vi "neo_sebesseg.vi"(7 "Jobb":dbl(slide) scale=-5.0..5.0, 8 "error in (no error)":errorcluster, 9 "Bal":dbl(slide) scale=-5.0..5.0, 10 "new reference in":refnum<k24>) -> (0 "error out":errorcluster, 2 "vissza":bool, 3 ".NET Refnum out":refnum<k24>)   [LabVIEW 2012]
uses:
  RosBridgeDotNet.dll
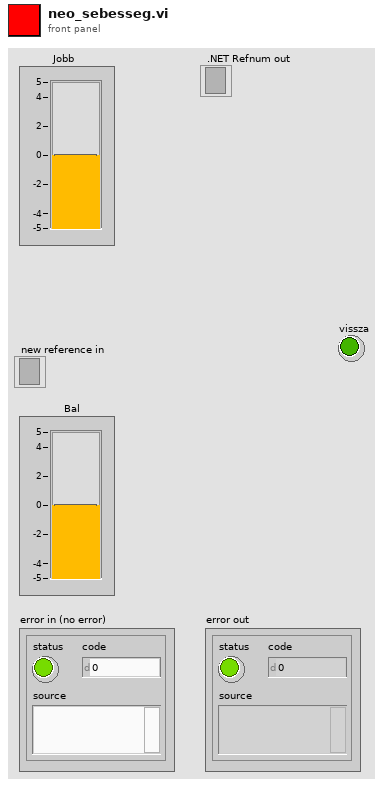
[diagram p1: front panel]
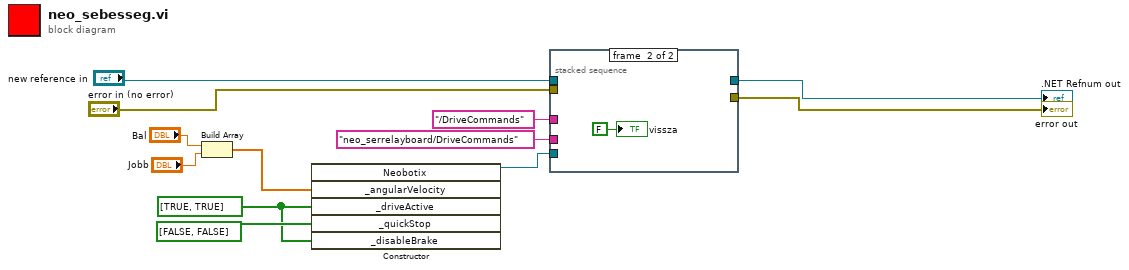
[diagram p0: block diagram]
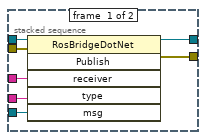
[diagram p2: hidden frame]
diagram:
  w8 = bool[] [TRUE, TRUE] ("_driveActive")
  n1 = Build Array("Bal", "Jobb") -> (w10:dbl[])
  n2 = constructor class="RosBridgeDotNet+Neobotix"("_angularVelocity"=w10, "_driveActive"=w8, "_quickStop"=bool[] [FALSE, FALSE] ("_driveActive"), "_disableBrake"=w8) -> (reference out=w3:refnum<k24>)  [unwired: 3 in, 6 out]
  n3 = stacked-sequence {
    tunnel: "/DriveCommands" ("receiver") -> [w19 _]
    tunnel: "neo_serrelayboard/DriveCommands" ("type") -> [w18 _]
    tunnel: w3 -> [w17 _]
    tunnel: "error in (no error)" -> [w16 _]
    tunnel: [w15 _] -> w7
    tunnel: [w14 _] -> w6
    tunnel: "new reference in" -> [w13 _]
    frame #0 {
      n4 = invoke class="RosBridgeDotNet" method="Publish"(reference=w13, error in=w16, "receiver"=w19, "type"=w18, "msg"=w17) -> (reference out=w14:refnum<k24>, error out=w15:errorcluster)  [unwired: 1 in, 4 out]
    }
    frame #1 {
      "vissza" <- FALSE ("Message 2")
    }
  }
  "error out" <- w7
  ".NET Refnum out" <- w6
